vi "AtSpectrograph_getEvent_gwState.vi"(8 "error in (no error)":errorcluster, 11 "logevent_gwState_Ctl":T1) -> (0 "error out":errorcluster, 2 "function return":i32, 3 "logevent_gwState_Ctl out":T1)   [LabVIEW 2016, in "SALLV_AtSpectrograph.lvlib"]
doc: "int AtSpectrograph_shm_getEvent_gwStateLV(AtSpectrograph_logevent_gwStateLV *logevent_gwState_Ctl );"
uses:
  SALLV_AtSpectrograph.lvlib
  DataTypes/logevent_gwState.ctl
  SALLV_AtSpectrograph.so
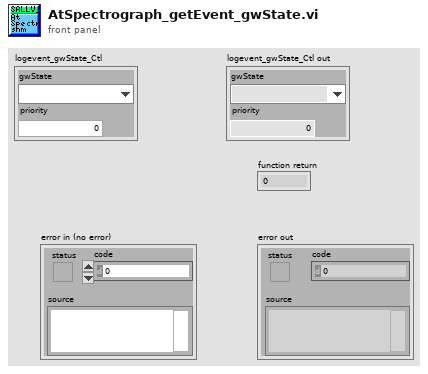
[diagram p1: front panel]
types:
  T1 = typedef "SALLV_AtSpectrograph.lvlib/logevent_gwState.ctl" = cluster{"gwState":enum32{"", "GwStationaryState", "GwMovingState"}, "priority":i32}
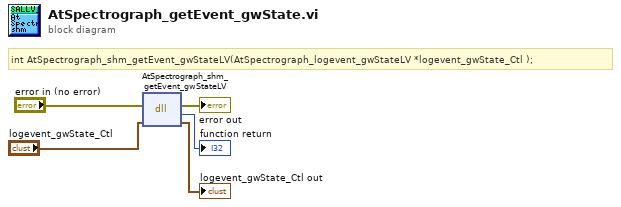
[diagram p0: block diagram]
diagram:
  # "int AtSpectrograph_shm_getEvent_gwStateLV(AtSpectrograph_logevent_gwStateLV *logevent_gwState_Ctl );"
  n1 = dll-call lib="home/harini/tcs/temp/SALLV_AtSpectrograph/SALLV_AtSpectrograph.*" fn="AtSpectrograph_shm_getEvent_gwStateLV"(error in="error in (no error)", "logevent_gwState_Ctl"="logevent_gwState_Ctl") -> (error out=→"error out":errorcluster, →"function return":i32, "logevent_gwState_Ctl"=→"logevent_gwState_Ctl out":T1)  [unwired: 2 in, 1 out]
